vi "util_clean_string.vi"(11 "string":string) -> (3 "string_clean":string)   [LabVIEW 2015, in "lv-builder-default.lvlib"]
uses:
  lv-builder-default.lvlib
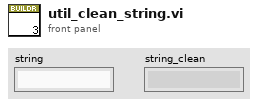
[diagram p1: front panel]
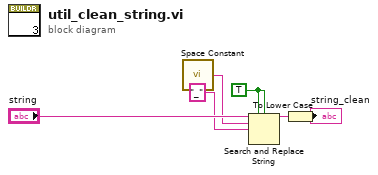
[diagram p0: block diagram]
diagram:
  w1 = TRUE ("replace all? (F)")
  n1 = call <vilib>:"Space Constant.vi"() -> ("String"=w4:string)
  n2 = Search and Replace String(replace all?=w1, case sensitive?=w1, input string="string", search string=w4, replace string="_" ("search string")) -> (result string=w3:string)  [unwired: 3 in, 3 out]
  n3 = To Lower Case(string=w3) -> (all lower case string=→"string_clean":string)
